vi "Configure Trigger Event Digital IO.vi"(0 "VISA resource name":refnum<visa-resource-name>, 1 "Trigger Pulse Width (1E-6 S)":dbl=1e-06, 5 "Trigger Number (1)":i32=1, 7 "Trigger Mode (0: Bypass)":i32(ring) items=["Bypass", "Falling Edge", "Rising Edge", "Falling and Rising Edge", "Synchronous-A", "Synchronous", "Synchronous-M", "Rising-A", "Rising-M"], 9 "Event ID":string, 11 "error in (no error)":errorcluster) -> (4 "VISA resource name out":refnum<visa-resource-name>, 15 "error out":errorcluster)   [LabVIEW 2019, in "Keithley 2600 Series.lvlib"]
doc: "Configures the event that causes a trigger to be asserted on the digital output line.\n\n<b>Notes:</b>\n(1) This VI is not available on the models 2604B, 2614B, and 2634B.\n(2) In order to allow for the configuration to achieve a known default state, it's required to call <b>Reset Trigger Event</b> VI before you call this VI."
uses:
  Keithley 2600 Series.lvlib
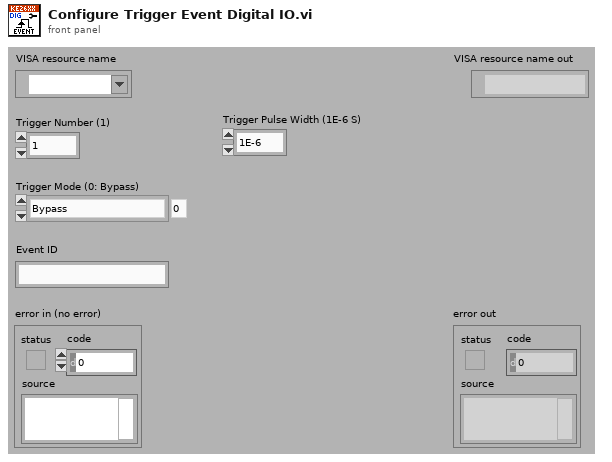
[diagram p1: front panel]
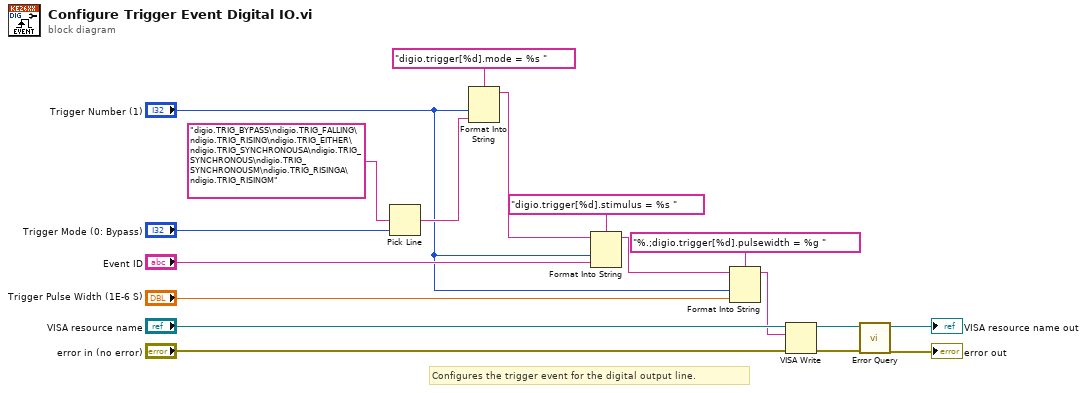
[diagram p0: block diagram]
diagram:
  # "Configures the trigger event for the digital output line."
  n1 = Pick Line(multi-line string="digio.TRIG_BYPASS\ndigio.TRIG_FALLING\ndigio.TRIG_RISING\ndigio.TRIG_EITHER\ndigio.TRIG_SYNCHRONOUSA\ndigio.TRIG_SYNCHRONOUS\ndigio.TRIG_SYNCHRONOUSM\ndigio.TRIG_RISINGA\ndigio.TRIG_RISINGM", line index="Trigger Mode (0: Bypass)") -> (output string=w15:string)  [unwired: 1 in]
  n2 = Format Into String(format string="digio.trigger[%d].mode = %s ", "Trigger Number (1)", w15) -> (resulting string=w14:string)  [unwired: 2 in, 1 out]
  n3 = Format Into String(format string="digio.trigger[%d].stimulus = %s ", initial string=w14, "Trigger Number (1)", "Event ID") -> (resulting string=w4:string)  [unwired: 1 in, 1 out]
  n4 = Format Into String(format string="%.;digio.trigger[%d].pulsewidth = %g ", initial string=w4, "Trigger Number (1)", "Trigger Pulse Width (1E-6 S)") -> (resulting string=w1:string)  [unwired: 1 in, 1 out]
  n5 = VISA Write(VISA resource name="VISA resource name", write buffer=w1, error in (no error)="error in (no error)") -> (VISA resource name out=w9:refnum<visa-resource-name>, error out=w8:errorcluster)  [unwired: 1 out]
  n6 = call "Error Query.vi"("error in (no error)"=w8, "VISA resource name"=w9) -> ("error out"=→"error out":errorcluster, "VISA resource name out"=→"VISA resource name out":refnum<visa-resource-name>)  [unwired: 6 in, 2 out]
